vi "AutoAlign_P612.vi"() -> ()   [LabVIEW 2011]
uses:
  Controls/GraphNotifier2D.ctl
  Controls/StageStates.ctl
  <vilib>/LabVIEW Interface for Arduino/LabVIEW Interface for Arduino.lvlib
panel:
  out "Aligned":bool
  in  "Repeat":bool
  in  "Start":bool
  out "Intensity Graph":sgl[][](graph)
  in  "Quit":bool
  out "Sample":cluster{"X":dbl, "Y":dbl}[](graph)
  in  "Accumulations":i32=10
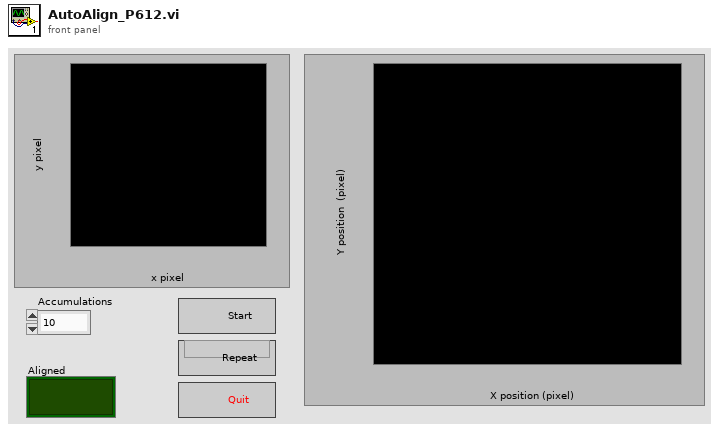
[diagram p1: front panel]
types:
  T1 = typedef "GraphNotifier2D.ctl" = cluster{"Xpos":i32, "Ypos":i32, "subarray":sgl[][], "Intensity":sgl}
  T2 = typedef "LabVIEW Interface for Arduino.lvlib/Arduino Resource.ctl" = cluster{"VISA resource":refnum<visa-resource-name>, "Board Type":T3, "Connection Type":enum8{"USB / Serial"}, "Bytes Per Packet (15)":u8}
  T3 = typedef "LabVIEW Interface for Arduino.lvlib/Board Type.ctl" = enum16{"Uno", "Dimuelanove w/Atmega 328", "Mega 2560"}
  T4 = typedef "StageStates.ctl" = enum16{"POSITION", "MVR", "MOVE", "HALT", "ONTARGET", "ERROR", "EXIT", "HOME", "ZEROPOS", "NANOPOS", "QUIT", "ANALOG"}
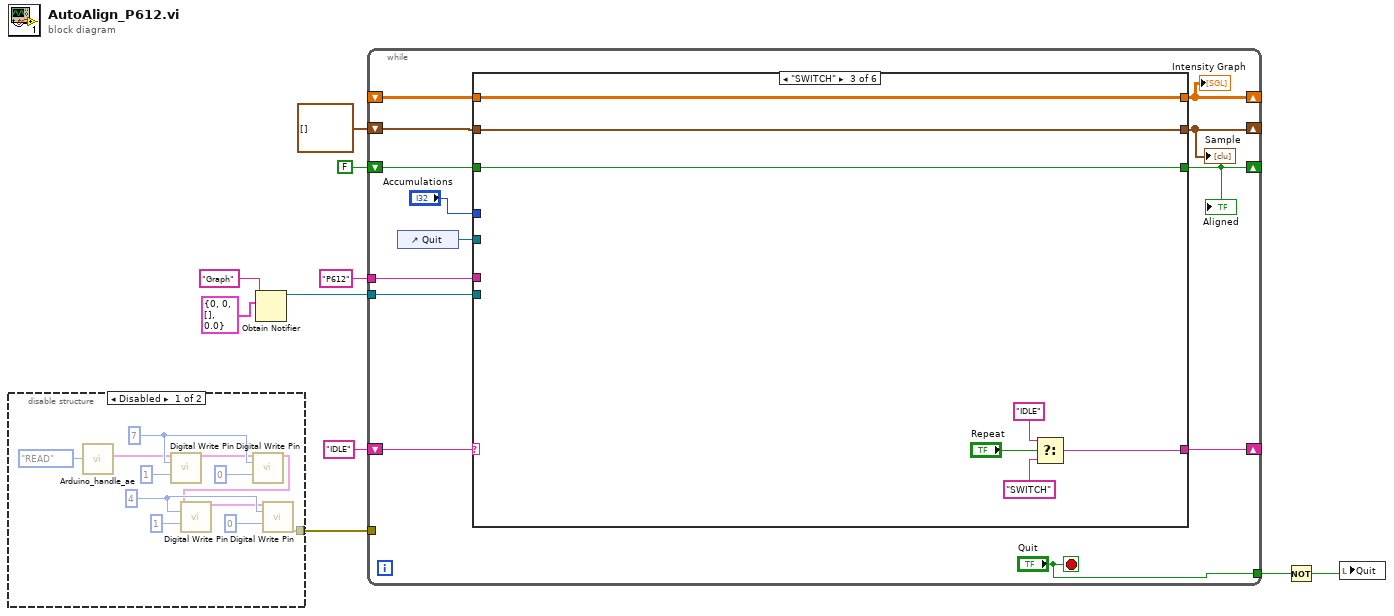
[diagram p0: block diagram]
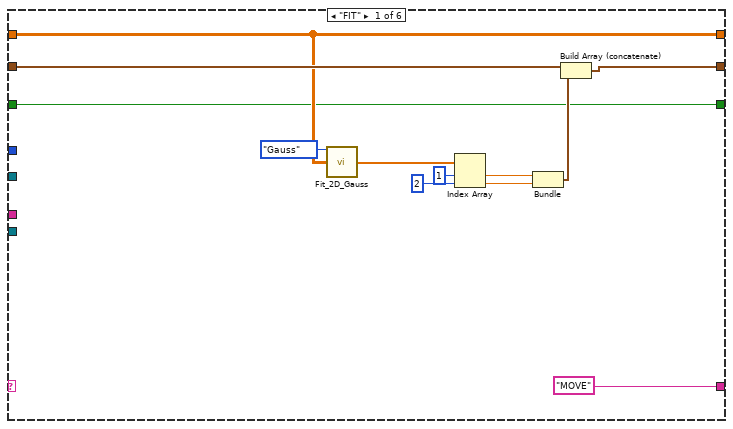
[diagram p3: hidden frame]
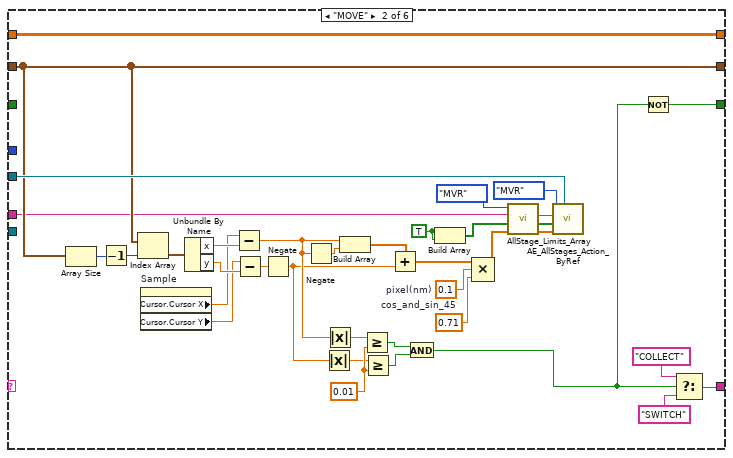
[diagram p4: hidden frame]
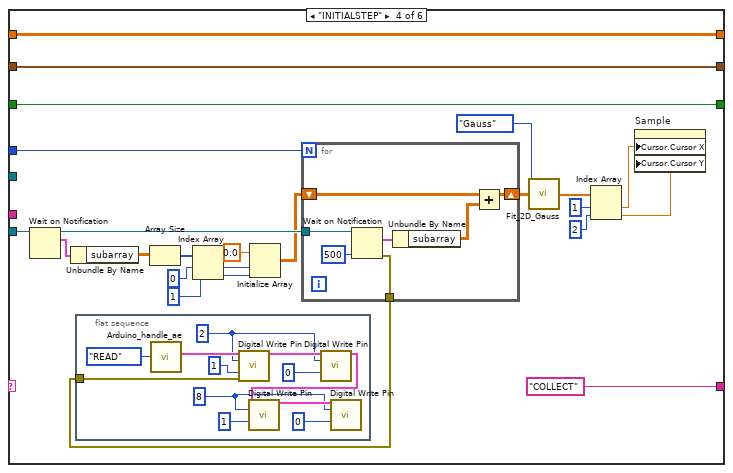
[diagram p5: hidden frame]
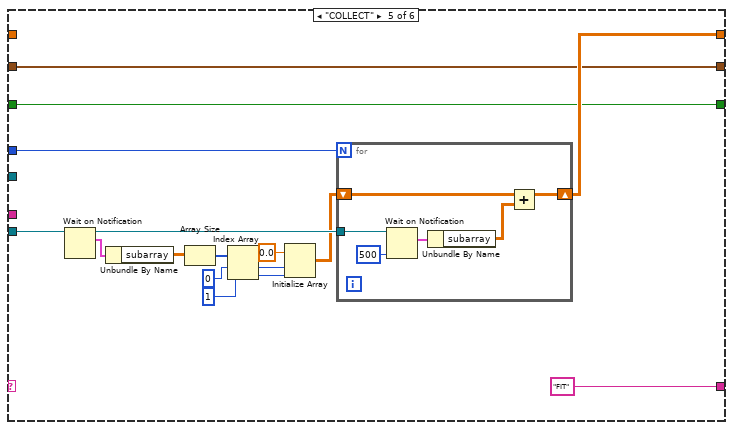
[diagram p6: hidden frame]
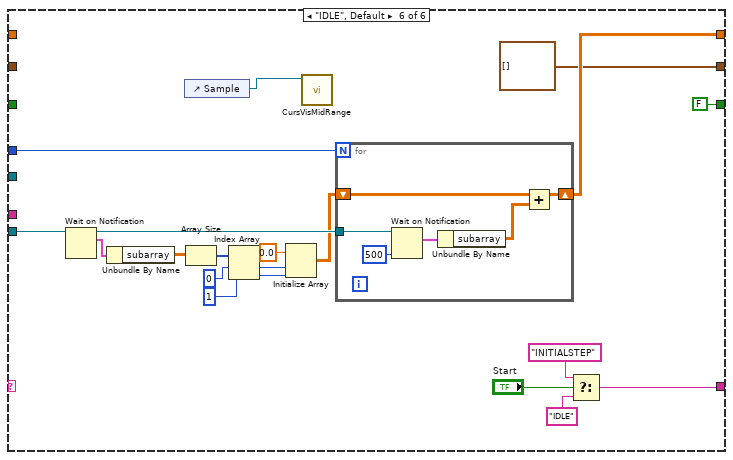
[diagram p7: hidden frame]
diagram:
  n1 = disable-structure shown="Disabled" {
    disable-tunnel: [w11 _] -> w6
    frame Disabled {
      w22 = u8 4 ("Digital I/O Pin (0)")
      w17 = u8 7 ("Digital I/O Pin (0)")
      n2 = call "Arduino_handle_ae.vi"("Enum"=enum16{"WRITE", "READ"}."READ") -> ("Arduino Resource Out"=w16:T2)  [unwired: 10 in]
      n3 = call <vilib>:"Digital Write Pin.vi"("Arduino Resource"=w16, "Digital I/O Pin (0)"=w17, "Value (0)"=u8 1) -> ("Arduino Resource"=w12:T2)  [unwired: 11 in, 1 out]
      n4 = call <vilib>:"Digital Write Pin.vi"("Arduino Resource"=w12, "Digital I/O Pin (0)"=w17, "Value (0)"=u8 0) -> ("Arduino Resource"=w21:T2)  [unwired: 11 in, 1 out]
      n5 = call <vilib>:"Digital Write Pin.vi"("Arduino Resource"=w21, "Digital I/O Pin (0)"=w22, "Value (0)"=u8 1) -> ("Arduino Resource"=w20:T2)  [unwired: 11 in, 1 out]
      n6 = call <vilib>:"Digital Write Pin.vi"("Arduino Resource"=w20, "Digital I/O Pin (0)"=w22, "Value (0)"=u8 0) -> ("error out"=w11:errorcluster)  [unwired: 11 in, 1 out]
    }
    frame Enabled {
    }
  }
  n7 = Obtain Notifier(name (unnamed)="Graph", notification data type=T1 {"Xpos"=0, "Ypos"=0, "subarray"=[], "Intensity"=0.0}) -> (notifier out=w3:refnum<notifier>)  [unwired: 2 in, 2 out]
  n8 = while {
    shift-right: [w33] -> _
    shift-left: _ -> [w35]
    shift-right: [w34] -> _
    shift-left: cluster{"x":dbl, "y":dbl}[] [] ("XY chart data") -> [w24]
    shift-right: [w32] -> _
    shift-left: "IDLE" -> [w28]
    shift-right: [w30] -> _
    shift-left: FALSE -> [w31]
    tunnel: w3 -> [w27]
    tunnel: "P612" ("StageID") -> [w25]
    tunnel: w6 -> [_]
    tunnel: ["Quit"] -> w2
    stop <- "Quit" stop-if-true
    n9 = control-ref of="Quit"() -> (w29:refnum<vi>)
    n10 = case shown="\"SWITCH\"" w28 {
      tunnel: [w43 w84 w89 w115 w150 w176] -> w33
      tunnel: w35 -> [w43 w84 w89 w115 _ _]
      tunnel: w24 -> [w45 w57 w90 w112 w149 _]
      tunnel: [w44 w57 w90 w112 w149 cluster{"x":dbl, "y":dbl}[] [] ("XY chart data")] -> w34
      tunnel: w25 -> [_ w50 _ _ _ _]
      tunnel: ["MOVE" w70 w86 "COLLECT" "FIT" w174] -> w32
      tunnel: w31 -> [w41 _ w91 w114 w148 _]
      tunnel: [w41 w55 w91 w114 w148 FALSE] -> w30
      tunnel: w29 -> [_ w75 _ _ _ _]
      tunnel: w27 -> [_ _ _ w100 w137 w167]
      tunnel: "Accumulations" -> [_ _ _ w101 w146 w171]
      frame "FIT" {
        n11 = call "Fit_2D_Gauss.vi"("Enum"=enum16{"Gauss", "Lorentz"}."Gauss", "Image IN"=w43) -> ("Fit Parameters"=w47:dbl[])  [unwired: 12 in, 1 out]
        n12 = Index Array(array=w47, index #1=1 ("index"), index #2=2 ("index")) -> (element #1=w38:dbl, element #2=w37:dbl)
        n13 = Bundle("Numeric"=w38, "Numeric"=w37) -> (w46:cluster{"Numeric":dbl, "Numeric":dbl})  [unwired: 1 in]
        n14 = Build Array (concatenate)(w45, w46) -> (w44:cluster{"Numeric":dbl, "Numeric":dbl}[])
      }
      frame "MOVE" {
        w69 = 0.71  # cos_and_sin_45
        w83 = 0.01 ("y")
        w82 = 0.1  # pixel(nm)
        w81 = TRUE
        n15 = Array Size(array=w57) -> (size(s)=w76:i32)
        n16 = Decrement(x=w76) -> (x-1=w68:i32)
        n17 = Index Array(array=w57, index=w68) -> (element=w77:cluster{"x":dbl, "y":dbl})
        n18 = property on="Sample" class="XYGraph (strict)"() -> ("Cursor.Cursor X"=w74:dbl, "Cursor.Cursor Y"=w73:dbl)  [unwired: 2 in, 2 out]
        n19 = Unbundle By Name(w77) -> ("x"=w78:dbl, "y"=w79:dbl)
        n20 = Subtract(x=w74, y=w78) -> (x-y=w64:dbl)
        n21 = Subtract(x=w73, y=w79) -> (x-y=w65:dbl)
        n22 = Negate(x=w65) -> (-x=w61:dbl)
        n23 = Negate(x=w64) -> (-x=w63:dbl)
        n24 = Absolute Value(x=w61) -> (abs(x)=w66:dbl)
        n25 = Absolute Value(x=w64) -> (abs(x)=w67:dbl)
        n26 = Build Array(w64, w63) -> (w62:dbl[])
        n27 = Greater Or Equal?(x=w67, y=w83) -> (x >= y?=w59:bool)
        n28 = Greater Or Equal?(x=w66, y=w83) -> (x >= y?=w58:bool)
        n29 = Add(x=w62, y=w61) -> (x+y=w60:dbl[])
        n30 = And(x=w59, y=w58) -> (x .and. y?=w56:bool)
        n31 = Build Array(w81, w81) -> (w49:bool[])
        n32 = Compound Arithmetic op=MULTIPLY(w60, w82, w69) -> (w51:dbl[])
        n33 = call "AllStage_Limits_Array.vi"("Step(um)/Position(units)"=w51, "Axis"=w49, "Stage ID"=w50, "MOVE/MVR"=enum16{"MOVE", "MVR"}."MVR") -> ("Positions"=w52:dbl[], "Boolean Array"=w53:bool[], "Stage ID"=w54:string)  [unwired: 5 in]
        n34 = call "AE_AllStages_Action_ByRef.vi"("Abort"=w75, "Positions"=w52, "Axis"=w53, "Stage ID"=w54, "Action"=StageStates."MVR") -> ()  [unwired: 3 in, 4 out]
        n35 = Not(x=w56) -> (.not. x?=w55:bool)
        n36 = Select(t="COLLECT", s=w56, f="SWITCH") -> (s? t:f=w70:string)
      }
      frame "SWITCH" {
        n37 = Select(t="IDLE", s="Repeat", f="SWITCH") -> (s? t:f=w86:string)
      }
      frame "INITIALSTEP" {
        n38 = Wait on Notification(notifier=w100) -> (notifier out=w103:refnum<notifier>, notification=w111:T1)  [unwired: 3 in, 2 out]
        n39 = Unbundle By Name(w111) -> ("subarray"=w110:sgl[][])
        n40 = flat-sequence {
          tunnel: w99 -> [w116]
          frame #0 {
            w117 = u8 8 ("Digital I/O Pin (0)")
            w122 = u8 2 ("Digital I/O Pin (0)")
            n41 = call "Arduino_handle_ae.vi"("Enum"=enum16{"WRITE", "READ"}."READ") -> ("Arduino Resource Out"=w123:T2)  [unwired: 10 in]
            n42 = call <vilib>:"Digital Write Pin.vi"("Arduino Resource"=w123, "Digital I/O Pin (0)"=w122, "Value (0)"=u8 1, "error in"=w116) -> ("Arduino Resource"=w127:T2)  [unwired: 10 in, 1 out]
            n43 = call <vilib>:"Digital Write Pin.vi"("Arduino Resource"=w127, "Digital I/O Pin (0)"=w122, "Value (0)"=u8 0) -> ("Arduino Resource"=w118:T2)  [unwired: 11 in, 1 out]
            n44 = call <vilib>:"Digital Write Pin.vi"("Arduino Resource"=w118, "Digital I/O Pin (0)"=w117, "Value (0)"=u8 1) -> ("Arduino Resource"=w119:T2)  [unwired: 11 in, 1 out]
            n45 = call <vilib>:"Digital Write Pin.vi"("Arduino Resource"=w119, "Digital I/O Pin (0)"=w117, "Value (0)"=u8 0) -> ()  [unwired: 11 in, 2 out]
          }
        }
        n46 = Array Size(array=w110) -> (size(s)=w109:i32[])
        n47 = Index Array(array=w109, index #1=0 ("index"), index #2=1 ("index")) -> (element #1=w106:i32, element #2=w105:i32)
        n48 = Initialize Array(sgl 0.0 ("element"), w106, w105) -> (w102:sgl[][])
        n49 = for {
          N: w101 -> [_]
          shift-right: [w134] -> w95
          shift-left: w102 -> [w133]
          tunnel: w103 -> [w131]
          tunnel: [w128] -> w99
          n50 = Wait on Notification(notifier=w131, timeout in ms (-1)=500) -> (notification=w130:T1, error out=w128:errorcluster)  [unwired: 2 in, 2 out]
          n51 = Unbundle By Name(w130) -> ("subarray"=w129:sgl[][])
          n52 = Add(x=w133, y=w129) -> (x+y=w134:sgl[][])
        }
        n53 = call "Fit_2D_Gauss.vi"("Enum"=enum16{"Gauss", "Lorentz"}."Gauss", "Image IN"=w95) -> ("Fit Parameters"=w98:dbl[])  [unwired: 12 in, 1 out]
        n54 = Index Array(array=w98, index #1=1 ("index"), index #2=2 ("index")) -> (element #1=w94:dbl, element #2=w93:dbl)
        n55 = property on="Sample" class="XYGraph (strict)"("Cursor.Cursor X"=w94, "Cursor.Cursor Y"=w93) -> ()  [unwired: 2 in, 2 out]
      }
      frame "COLLECT" {
        n56 = Wait on Notification(notifier=w137) -> (notifier out=w136:refnum<notifier>, notification=w145:T1)  [unwired: 3 in, 2 out]
        n57 = Unbundle By Name(w145) -> ("subarray"=w144:sgl[][])
        n58 = Array Size(array=w144) -> (size(s)=w143:i32[])
        n59 = Index Array(array=w143, index #1=0 ("index"), index #2=1 ("index")) -> (element #1=w140:i32, element #2=w139:i32)
        n60 = Initialize Array(sgl 0.0 ("element"), w140, w139) -> (w135:sgl[][])
        n61 = for {
          N: w146 -> [_]
          shift-right: [w156] -> w150
          shift-left: w135 -> [w155]
          tunnel: w136 -> [w153]
          n62 = Wait on Notification(notifier=w153, timeout in ms (-1)=500) -> (notification=w152:T1)  [unwired: 2 in, 3 out]
          n63 = Unbundle By Name(w152) -> ("subarray"=w151:sgl[][])
          n64 = Add(x=w155, y=w151) -> (x+y=w156:sgl[][])
        }
      }
      frame "IDLE", Default {
        n65 = Wait on Notification(notifier=w167) -> (notifier out=w166:refnum<notifier>, notification=w169:T1)  [unwired: 3 in, 2 out]
        n66 = Unbundle By Name(w169) -> ("subarray"=w168:sgl[][])
        n67 = control-ref of="Sample"() -> (w158:refnum<vi>)
        n68 = Array Size(array=w168) -> (size(s)=w165:i32[])
        n69 = Index Array(array=w165, index #1=0 ("index"), index #2=1 ("index")) -> (element #1=w162:i32, element #2=w161:i32)
        n70 = Initialize Array(sgl 0.0 ("element"), w162, w161) -> (w159:sgl[][])
        n71 = call "CursVisMidRange.vi"("XYGraph in"=w158) -> ()  [unwired: 11 in]
        n72 = for {
          N: w171 -> [_]
          shift-right: [w182] -> w176
          shift-left: w159 -> [w181]
          tunnel: w166 -> [w179]
          n73 = Wait on Notification(notifier=w179, timeout in ms (-1)=500) -> (notification=w178:T1)  [unwired: 2 in, 3 out]
          n74 = Unbundle By Name(w178) -> ("subarray"=w177:sgl[][])
          n75 = Add(x=w181, y=w177) -> (x+y=w182:sgl[][])
        }
        n76 = Select(t="INITIALSTEP", s="Start", f="IDLE") -> (s? t:f=w174:string)
      }
    }
    "Sample" <- w34
    "Intensity Graph" <- w33
    "Aligned" <- w30
  }
  n77 = Not(x=w2) -> (.not. x?=w1:bool)
  n78 = local write "Quit"(w1) -> ()
